vi "Test Weight Grab and Apply.vi"() -> ()   [LabVIEW 2011]
uses:
  GrabberTool Class.lvclass
  WorkTable Class/WorkTable Class.lvclass
  Gantry Class/Gantry Class.lvclass
  Config Manager Class/Type Definitions/Fiducial Type.ctl
  CameraTool Class/Type Definitions/Fiducial Acquisition Parameters.ctl
  Config Manager Class/Type Definitions/Weight Type.ctl
  Orient3d Class/Orient3d Class.lvclass
  Vec3d Class/Vec3d Class.lvclass
  Utils/Type Definitions/Position_Orientation.ctl
  WorkTable Class/Type Definitions/Worktable_Weight.ctl
  CameraTool Class/CameraTool Class.lvclass
  Config Manager Class/Config Manager Class.lvclass
panel:
  out "error out":errorcluster
  in  "Apply Weight on Slot":i32
  in  "Apply Weight on Chuck":i32
  in  "Weight Slot":i32
  in  "Config Folder":path=path "C:/Users/husker/Desktop/gantry/Config"
  in  "Virtual Mode":bool
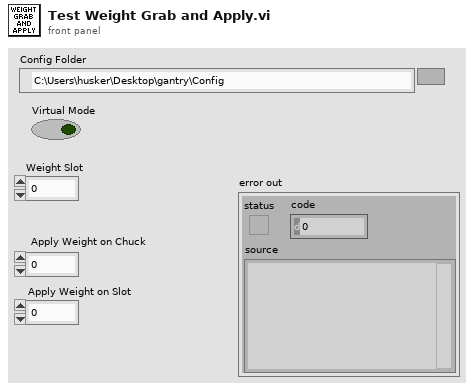
[diagram p1: front panel]
types:
  T1 = enum16{"Empty", "Bare HDI", "Unglued", "Stamped", "PartOnTop", "Weighted", "Unpotted", "Potted"}
  T2 = typedef "Worktable_Weight.ctl" = cluster{"Weight State":enum16{"Empty", "Populated"}, "Weight Type":T3, "Location/Orientation":T4}
  T3 = typedef "Weight Type.ctl" = enum16{"Weight 1", "Weight 2", "Weight 3", "Weight 4", "Weight 5", "Weight 6", "Weight 7", "Weight 8"}
  T4 = typedef "Position_Orientation.ctl" = cluster{"Center":refnum<class "Vec3d Class.lvclass">, "Orientation":refnum<class "Orient3d Class.lvclass">}
  T5 = typedef "Fiducial Type.ctl" = enum16{"HDI", "BBM"}
  T6 = typedef "Fiducial Acquisition Parameters.ctl" = cluster{"Selection Criteria":enum16{"Single", "Top", "Bottom"}, "Image Prefix":string, "Fiducial Type":T5}
  T7 = cluster{"Feature Coordinates":refnum<class "Vec3d Class.lvclass">, "Feature Name":string}[]
  T8 = typedef "Fiducial Image.ctl" = cluster{"Fiducial Image":T9, "Selected Fiducial":T11, "fiducial name":string}
  T9 = typedef "Physical Image.ctl" = cluster{"Image Position":refnum<class "Vec3d Class.lvclass">, "Image Reference":T10, "Field of View":cluster{"x(mm)":dbl, "y(mm)":dbl}}
  T10 = typedef "IMAQ Image.ctl" = refnum<image>
  T11 = typedef "Fiducial with Source.ctl" = cluster{"Fiducial Image Coordinate":refnum<class "Vec3d Class.lvclass">, "Fiducial Source":enum16{"Pattern Recognition", "User", "Error", "Default"}}
  T12 = typedef "Worktable_Module Slot.ctl" = cluster{"Slot State":enum16{"Empty", "Bare HDI", "Unglued", "Stamped", "PartOnTop", "Weighted", "Unpotted", "Potted"}, "BBM Type":enum16{"None", "BBM", "GlassSlide"}, "HDI Type":enum16{"None", "HDI", "Polyimide"}, "Vacuum Channel":u8, "Location/Orientation BBM":T4, "Location/Orientation HDI":T4, "S/N":string}
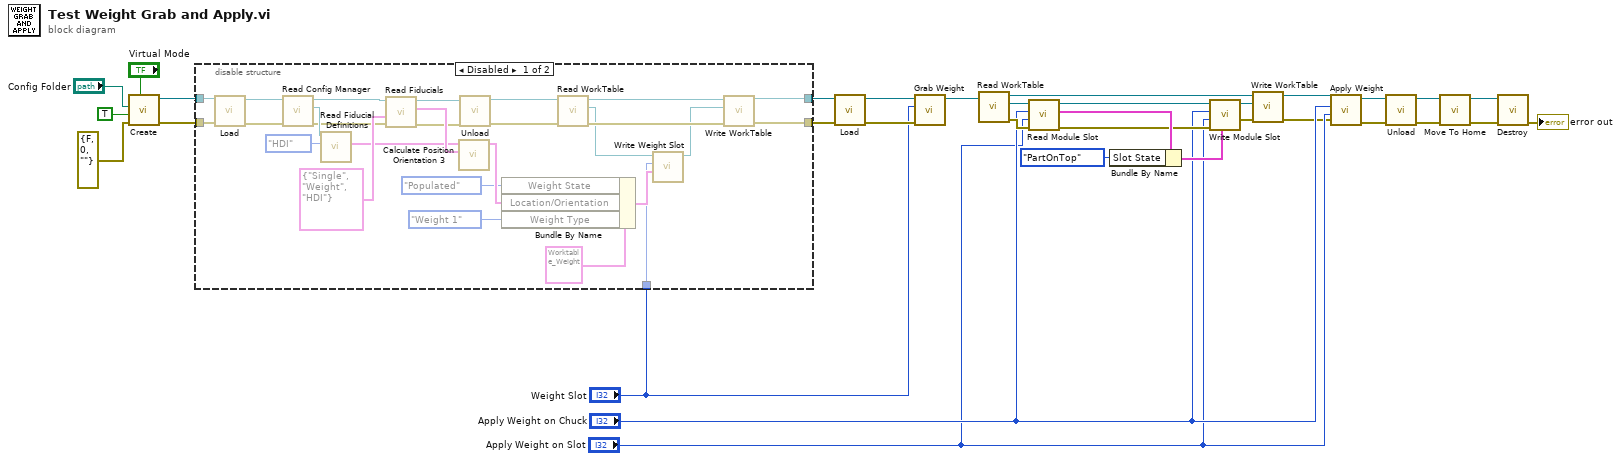
[diagram p0: block diagram]
diagram:
  n1 = call "Create.vi"("Virtual Mode"="Virtual Mode", "error in"=errorcluster {"status"=FALSE, "code"=0, "source"=""}, "HOME?"=TRUE, "Config Folder"="Config Folder") -> ("error out"=w17:errorcluster, "Gantry out"=w18:refnum<class "Gantry Class.lvclass">)  [unwired: 6 in]
  n2 = disable-structure shown="Disabled" {
    disable-tunnel: w18 -> [w60 w62]
    disable-tunnel: w17 -> [w49 w61]
    disable-tunnel: [w40 w62] -> w20
    disable-tunnel: [w39 w61] -> w19
    disable-tunnel: "Weight Slot" -> [w34 _]
    frame Disabled {
      n3 = call "Load.vi"("error in"=w49, "Gantry In"=w60) -> ("error out"=w48:errorcluster, "CameraTool out"=w55:refnum<class "CameraTool Class.lvclass">)  [unwired: 8 in]
      n4 = call-dynamic "Read Config Manager.vi"("error in"=w48, "Gantry in"=w55) -> ("error out"=w47:errorcluster, "Config Manager"=w54:refnum<class "Config Manager Class.lvclass">, "Gantry out"=w53:refnum<class "CameraTool Class.lvclass">)  [unwired: 7 in]
      n5 = call "Read Fiducial Definitions.vi"("Fiducial Type"=Fiducial_Type."HDI", "Config Manager in"=w54) -> ("Feature Definitions"=w57:T7)  [unwired: 7 in, 2 out]
      n6 = call-dynamic "Read Fiducials.vi"("error in"=w47, "Fiducial Acquisition Parameters"=T6 {"Selection Criteria"=enum."Single", "Image Prefix"="Weight", "Fiducial Type"=enum."HDI"}, "CameraTool in"=w53) -> ("error out"=w46:errorcluster, "Fiducials"=w58:T8[], "CameraTool out"=w52:refnum<class "CameraTool Class.lvclass">)  [unwired: 6 in]
      n7 = call "Calculate Position Orientation 3.vi"("Fiducials"=w58, "Feature Definitions"=w57) -> ("PositionOrientation"=w50:T4)  [unwired: 8 in, 1 out]
      n8 = call "Unload.vi"("error in"=w46, "CameraTool in"=w52) -> ("error out"=w37:errorcluster, "Gantry out"=w38:refnum<class "Gantry Class.lvclass">)  [unwired: 8 in]
      n9 = Bundle By Name(cluster=T2 {"Weight State"=enum."Empty", "Weight Type"=enum."Weight 1", "Location/Orientation"={"Center"=refnum, "Orientation"=refnum}} ("Weight Slot"), "Weight State"=enum16{"Empty", "Populated"}."Populated", "Location/Orientation"=w50, "Weight Type"=Weight_Type."Weight 1") -> (w35:T2)
      n10 = call-dynamic "Read WorkTable.vi"("error in"=w37, "Gantry Class in"=w38) -> ("error out"=w45:errorcluster, "WorkTable Class.lvclass"=w44:refnum<class "WorkTable Class.lvclass">, "Gantry Class out"=w51:refnum<class "Gantry Class.lvclass">)  [unwired: 7 in]
      n11 = call "Write Weight Slot.vi"("Weight Slot"=w35, "weight slot"=w34, "WorkTable Class in"=w44) -> ("WorkTable Class out"=w43:refnum<class "WorkTable Class.lvclass">)  [unwired: 7 in, 1 out]
      n12 = call-dynamic "Write WorkTable.vi"("error in (no error)"=w45, "WorkTable Class.lvclass"=w43, "Gantry Class in"=w51) -> ("error out"=w39:errorcluster, "Gantry Class out"=w40:refnum<class "Gantry Class.lvclass">)  [unwired: 7 in]
    }
    frame Enabled {
    }
  }
  n13 = call "Load.vi"("error in"=w19, "Gantry In"=w20) -> ("error out"=w28:errorcluster, "Grabber Tool out"=w29:refnum<class "GrabberTool Class.lvclass">)  [unwired: 8 in]
  n14 = call "Grab Weight.vi"("error in"=w28, "Weight Number"="Weight Slot", "GrabberTool in"=w29) -> ("GrabberTool out"=w6:refnum<class "GrabberTool Class.lvclass">)  [unwired: 7 in, 1 out]
  n15 = call-dynamic "Read WorkTable.vi"("Gantry Class in"=w6) -> ("error out"=w14:errorcluster, "WorkTable Class.lvclass"=w15:refnum<class "WorkTable Class.lvclass">, "Gantry Class out"=w10:refnum<class "GrabberTool Class.lvclass">)  [unwired: 8 in]
  n16 = call-dynamic "Read Module Slot.vi"("error in"=w14, "slot"="Apply Weight on Slot", "chuck"="Apply Weight on Chuck", "WorkTable in"=w15) -> ("error out"=w11:errorcluster, "Module Slot"=w13:T12, "WorkTable out"=w9:refnum<class "WorkTable Class.lvclass">)  [unwired: 5 in]
  n17 = Bundle By Name(cluster=w13, "Slot State"=T1."PartOnTop") -> (w12:T12)
  n18 = call-dynamic "Write Module Slot.vi"("Module Slot"=w12, "error in"=w11, "slot"="Apply Weight on Slot", "chuck"="Apply Weight on Chuck", "WorkTable in"=w9) -> ("error out"=w7:errorcluster, "WorkTable out"=w8:refnum<class "WorkTable Class.lvclass">)  [unwired: 5 in]
  n19 = call-dynamic "Write WorkTable.vi"("error in (no error)"=w7, "WorkTable Class.lvclass"=w8, "Gantry Class in"=w10) -> ("error out"=w2:errorcluster, "Gantry Class out"=w3:refnum<class "GrabberTool Class.lvclass">)  [unwired: 7 in]
  n20 = call "Apply Weight.vi"("error in"=w2, "Slot Number"="Apply Weight on Slot", "Chuck Number"="Apply Weight on Chuck", "GrabberTool in"=w3) -> ("error out"=w26:errorcluster, "GrabberTool out"=w27:refnum<class "GrabberTool Class.lvclass">)  [unwired: 6 in]
  n21 = call "Unload.vi"("error in"=w26, "GrabberTool in"=w27) -> ("error out"=w24:errorcluster, "Gantry out"=w25:refnum<class "Gantry Class.lvclass">)  [unwired: 8 in]
  n22 = call-dynamic "Move To Home.vi"("error in"=w24, "Gantry in"=w25) -> ("error out"=w22:errorcluster, "Gantry out"=w23:refnum<class "Gantry Class.lvclass">)  [unwired: 8 in]
  n23 = call "Destroy.vi"("error in"=w22, "Gantry Class in"=w23) -> ("error out"=→"error out":errorcluster)  [unwired: 9 in]
